vi "HHSetSync.vi"(0 "SyncDiv":i32=1 min=1 max=8 step=1, 1 "CFD Level":i32=50 min=-1300 max=400 step=10, 2 "CFD ZeroX":i32=10 min=-1300 max=400 step=10, 3 "Offset":i32=10 min=-1300 max=400 step=10, 4 "DeviceIndex":i32) -> (5 "Error":bool)   [LabVIEW 2009]
uses:
  hhlib.dll
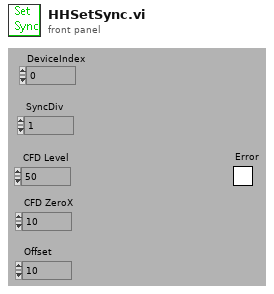
[diagram p1: front panel]
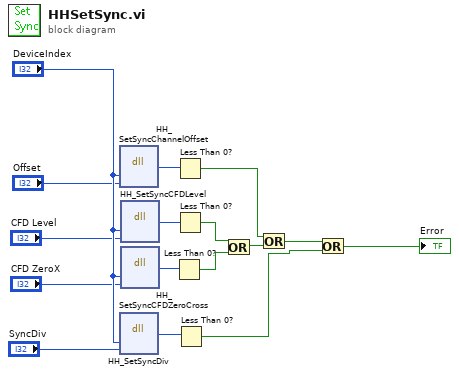
[diagram p0: block diagram]
diagram:
  n1 = dll-call lib="C:/Programme/Anwendungen/DAQLinescan_HH/hhlib.dll" fn="HH_SetSyncChannelOffset"("devidx"="DeviceIndex", "offset"="Offset") -> (w12:i32)  [unwired: 5 in, 2 out]
  n2 = dll-call lib="C:/Programme/Anwendungen/DAQLinescan_HH/hhlib.dll" fn="HH_SetSyncDiv"("devidx"="DeviceIndex", "divider"="SyncDiv") -> (w8:i32)  [unwired: 5 in, 2 out]
  n3 = dll-call lib="C:/Programme/Anwendungen/DAQLinescan_HH/hhlib.dll" fn="HH_SetSyncCFDLevel"("devidx"="DeviceIndex", "level"="CFD Level") -> (w11:i32)  [unwired: 5 in, 2 out]
  n4 = dll-call lib="C:/Programme/Anwendungen/DAQLinescan_HH/hhlib.dll" fn="HH_SetSyncCFDZeroCross"("devidx"="DeviceIndex", "Level"="CFD ZeroX") -> (w10:i32)  [unwired: 5 in, 2 out]
  n5 = Less Than 0?(x=w10) -> (x < 0?=w9:bool)
  n6 = Less Than 0?(x=w12) -> (x < 0?=w1:bool)
  n7 = Less Than 0?(x=w11) -> (x < 0?=w16:bool)
  n8 = Less Than 0?(x=w8) -> (x < 0?=w2:bool)
  n9 = Or(x=w16, y=w9) -> (x .or. y?=w15:bool)
  n10 = Or(x=w1, y=w15) -> (x .or. y?=w14:bool)
  n11 = Or(x=w14, y=w2) -> (x .or. y?=→"Error":bool)
